vi "MTMount_monitorCommand_setSimulationMode.vi"(8 "error in (no error)":errorcluster, 11 "command_setSimulationMode_Ctl":T1) -> (0 "error out":errorcluster, 2 "function return":i32, 3 "command_setSimulationMode_Ctl out":T1)   [LabVIEW 2018, in "SALLV_MTMount.lvlib"]
doc: "int MTMount_shm_monitorCommand_setSimulationModeLV(MTMount_command_setSimulationModeLV *command_setSimulationMode_Ctl );"
uses:
  SALLV_MTMount.lvlib
  DataTypes/command_setSimulationMode.ctl
  SALLV_MTMount.so
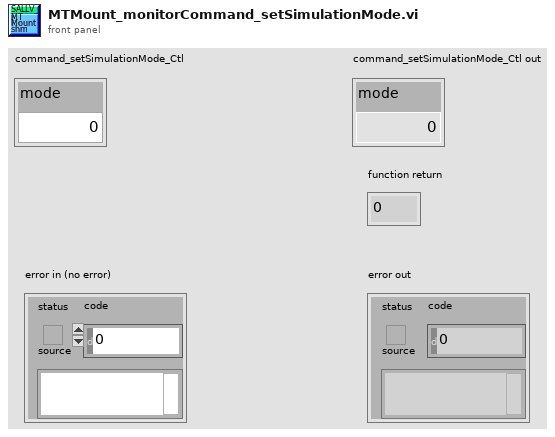
[diagram p1: front panel]
types:
  T1 = typedef "SALLV_MTMount.lvlib/command_setSimulationMode.ctl" = cluster{"mode":i32}
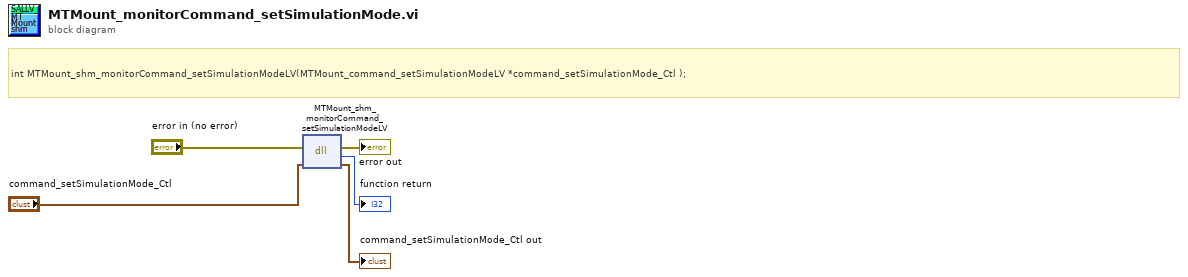
[diagram p0: block diagram]
diagram:
  # "int MTMount_shm_monitorCommand_setSimulationModeLV(MTMount_command_setSimulationModeLV *command_setSimulationMode_Ctl );"
  n1 = dll-call lib="home/ttsai/Document/salApiMTMount/SALLV_MTMount/SALLV_MTMount.*" fn="MTMount_shm_monitorCommand_setSimulationModeLV"(error in="error in (no error)", "command_setSimulationMode_Ctl"="command_setSimulationMode_Ctl") -> (error out=→"error out":errorcluster, →"function return":i32, "command_setSimulationMode_Ctl"=→"command_setSimulationMode_Ctl out":T1)  [unwired: 2 in, 1 out]
